vi "Interpolate XY-Points for Graphing.vi"(2 "Y":dbl[](array[numeric]) format="%_6g", 3 "X":dbl[](array[numeric]) format="%_6g") -> (0 "Y-Interpolated":dbl[](array[numeric]), 1 "X-Interpolated":dbl[](array[numeric]))   [LabVIEW 2016]
uses:
  <vilib>/gmath/NI_Gmath.lvlib
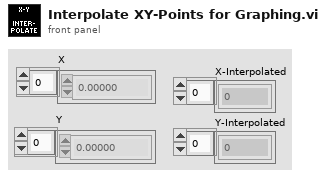
[diagram p1: front panel]
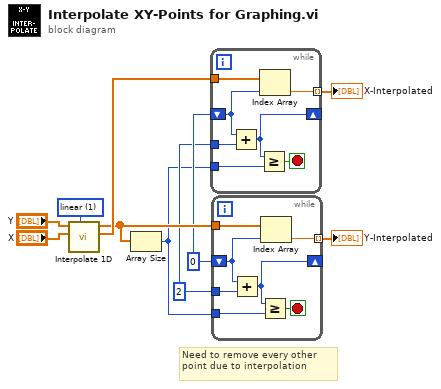
[diagram p0: block diagram]
diagram:
  w7 = 2 ("increment")
  w8 = 0 ("start index")
  w5 = 1 items=["nearest", "linear", "spline", "cubic Hermite", "Lagrange"] ("method")
  # "Need to remove every other point due to interpolation"
  n1 = call <vilib>:"Interpolate 1D.vi"("method"=w5, "X"="X", "Y"="Y") -> ("xi used"=w10:dbl[], "yi"=w9:dbl[])  [unwired: 6 in, 1 out]
  n2 = Array Size(array=w9) -> (size(s)=w6:i32)
  n3 = while "B-Field" {
    tunnel: w10 -> [w17]
    shift-right: [w14] -> _
    shift-left: w8 -> [w15]
    tunnel: [w16] -> w4 mode=indexing
    tunnel: w6 -> [w13]
    tunnel: w7 -> [w11]
    stop <- w12 stop-if-true
    n4 = Add(x=w15, y=w11) -> (x+y=w14:i32)
    n5 = Greater Or Equal?(x=w14, y=w13) -> (x >= y?=w12:bool)
    n6 = Index Array(array=w17, index=w15) -> (element=w16:dbl)
  }
  "X-Interpolated" <- w4
  n7 = while "In-Phase EPR Data" {
    tunnel: w9 -> [w24]
    shift-right: [w21] -> _
    shift-left: w8 -> [w22]
    tunnel: [w23] -> w3 mode=indexing
    tunnel: w7 -> [w20]
    tunnel: w6 -> [w19]
    stop <- w18 stop-if-true
    n8 = Add(x=w22, y=w20) -> (x+y=w21:i32)
    n9 = Greater Or Equal?(x=w21, y=w19) -> (x >= y?=w18:bool)
    n10 = Index Array(array=w24, index=w22) -> (element=w23:dbl)
  }
  "Y-Interpolated" <- w3
